vi "Subsystem.vi"(8 "Error In":errorcluster, 10 "Name":string, 11 "Channel In":refnum<class "Channel.lvclass">) -> (0 "Error Out":errorcluster, 3 "Channel Out":refnum<class "Channel.lvclass">)   [LabVIEW 2018, in "Toolkit.lvlib" / "Channel.lvclass"]
uses:
  Channel.lvclass
  Channel.lvclass/Channel.ctl
  Session/Session.lvclass/Session.ctl
  SSH/SSH.lvclass/SSH.ctl
  Session/Session.lvclass
  Toolkit.lvlib
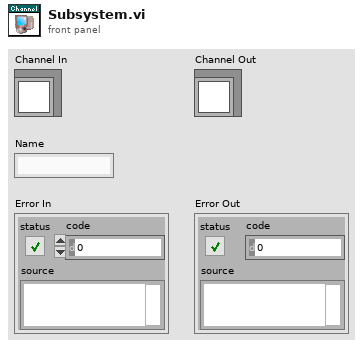
[diagram p1: front panel]
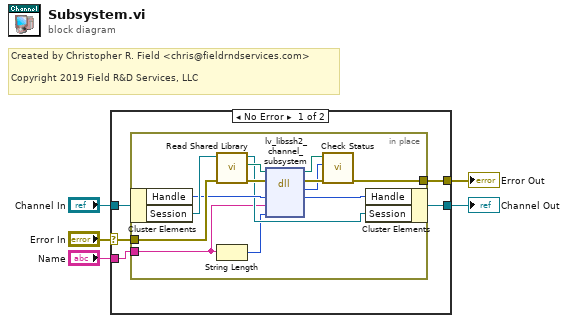
[diagram p0: block diagram]
diagram:
  # "Created by Christopher R. Field <chris@fieldrndservices.com>\n\nCopyright 2019 Field R&D Services, LLC"
  n1 = case shown="No Error" "Error In" {
    selector: "Error In" -> [w8 w25]
    tunnel: [w7 w25] -> w4
    tunnel: "Channel In" -> [w10 w24]
    tunnel: [w9 w24] -> w2
    tunnel: "Name" -> [w6 _]
    frame No Error {
      n2 = in-place {
        in-place-border: w8 -> [w20]
        in-place-border: [w16] -> w7
        in-place-border: w6 -> [w12]
        n3 = in-place-cluster #1(w10) -> ("Handle"=w15:u64, "Session"=w23:refnum<class "Session.lvclass">)
        n4 = call "Read Shared Library.vi"("Error In"=w20, "Session In"=w23) -> ("Erorr Out"=w21:errorcluster, "libssh2lv Shared Library"=w22:path, "Session Out"=w13:refnum<class "Session.lvclass">)  [unwired: 7 in]
        n5 = String Length(string=w12) -> (length=w11:i32)
        n6 = dll-call lib="libssh2lv.*" fn="lv_libssh2_channel_subsystem"(path in=w22, error in=w21, "handle"=w15, "subsystem"=w12, "subsystem_len"=w11) -> (path out=w18:path, error out=w19:errorcluster, "status"=w17:i32, "handle"=w14:u64)  [unwired: 3 in]
        n7 = call "Check Status.vi"("Error In"=w19, "Status"=w17, "lv-libssh2 Shared Library In"=w18) -> ("Error Out"=w16:errorcluster)  [unwired: 7 in, 1 out]
        n8 = in-place-cluster #1("Handle"=w14, "Session"=w13) -> (w9:refnum<class "Channel.lvclass">)
      }
    }
    frame Error {
    }
  }
  "Error Out" <- w4
  "Channel Out" <- w2
